vi "MyArchive.vi"(5 "archive filename":string, 6 "error in":errorcluster, 7 "archive mode":enum16{"direct", "append"}(ring), 8 "blocks to write":i32, 9 "ReadBuff refnum":refnum<file>) -> (0 "error out":errorcluster)   [LabVIEW 2013]
uses:
  My circular buffer info.ctl
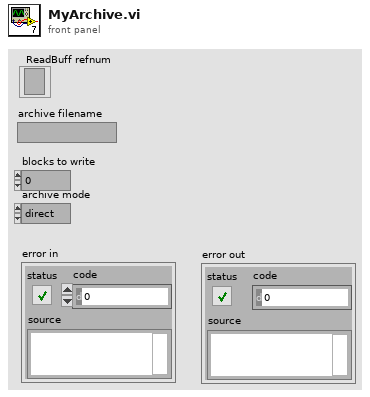
[diagram p1: front panel]
types:
  T1 = typedef "My circular buffer info.ctl" = cluster{"buff ref1":refnum<file>, "buff ref2":refnum<file>, "buffer1 path":path, "buffer2 path":path, "archive directory":path, "xml header":string, "num blocks  prior":i32, "num blocks after":i32, "blocks/event":i32, "samples/block":i32, "bytes/sample":i32, "number of channels":i32, "samples/block/channel":i32, "read buffer ref queue":refnum<queue>, "Event delay queue":refnum<queue>, "command queue":refnum<queue>}
  T2 = enum16{"open", "replace", "create", "open or create", "replace or create", "replace or create with confirmation"}
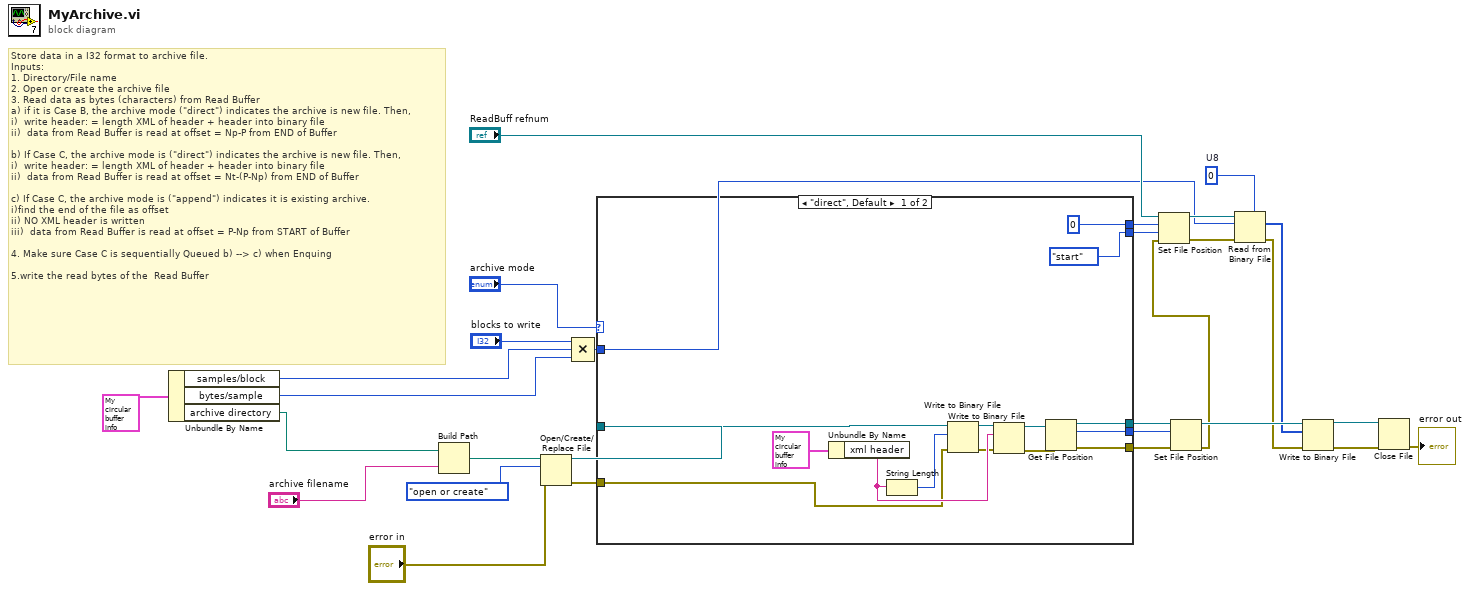
[diagram p0: block diagram]
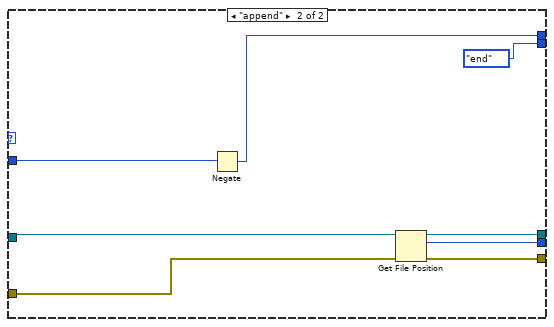
[diagram p2: hidden frame]
diagram:
  w16 = u8 0  # U8
  # "Store data in a I32 format to archive file.\nInputs:\n1. Directory/File name\n2. Open or create the archive file\n3. Read data as bytes (characters) from Read Buffer\na) if it is Case B, the archive mode (\"direct\") indicates the archive is new file. Then, \ni)  write header: = length XML of header + header into binary file\nii)  data from Read Buffer is read at offset = Np-P from END of Buffer\n\nb) If Case C, the archive mode is (\"direct\") indicates the archive is new file. Then, \ni)  write header: = length XML of header + header into binary file\nii)  data from Read Buffer is read at offset = Nt-(P-Np) from END of Buffer\n\nc) If Case C, the archive mode is (\"append\") indicates it is existing archive.  \ni)find the end of the file as offset\nii) NO XML header is written\niii)  data from Read Buffer is read at offset = P-Np from START of Buffer\n\n4. Make sure Case C is sequentially Queued b) --> c) when Enquing\n\n5.write the read bytes of the  Read Buffer"
  n1 = Unbundle By Name(T1 {"buff ref1"=refnum, "buff ref2"=refnum, "buffer1 path"=path "", "buffer2 path"=path "", "archive directory"=path "", "xml header"="", "num blocks  prior"=0, "num blocks after"=0, "blocks/event"=0, "samples/block"=0, "bytes/sample"=0, "number of channels"=0, "samples/block/channel"=0, "read buffer ref queue"=refnum, "Event delay queue"=refnum, "command queue"=refnum} ("My circular buffer info")) -> ("samples/block"=w22:i32, "bytes/sample"=w23:i32, "archive directory"=w28:path)
  n2 = Build Path(base path=w28, name or relative path="archive filename") -> (appended path=w26:path)
  n3 = Open/Create/Replace File(file path (use dialog)=w26, error in="error in", operation (0:open)=T2."open or create") -> (refnum out=w15:refnum<file>, error out=w7:errorcluster)  [unwired: 3 in, 1 out]
  n4 = Compound Arithmetic op=MULTIPLY("blocks to write", w22, w23) -> (w9:i32)
  n5 = case shown="\"direct\", Default" "archive mode" {
    tunnel: w9 -> [_ w51]
    tunnel: [0 w50] -> w20
    tunnel: [enum16{"start", "end", "current"}."start" ("from (0:start)") enum16{"start", "end", "current"}."end" ("from (0:start)")] -> w19
    tunnel: w15 -> [w41 w46]
    tunnel: [w36 w47] -> w14
    tunnel: [w35 w48] -> w13
    tunnel: w7 -> [w33 w45]
    tunnel: [w30 w44] -> w6
    frame "direct", Default {
      n6 = Unbundle By Name(T1 {"buff ref1"=refnum, "buff ref2"=refnum, "buffer1 path"=path "", "buffer2 path"=path "", "archive directory"=path "", "xml header"="", "num blocks  prior"=0, "num blocks after"=0, "blocks/event"=0, "samples/block"=0, "bytes/sample"=0, "number of channels"=0, "samples/block/channel"=0, "read buffer ref queue"=refnum, "Event delay queue"=refnum, "command queue"=refnum} ("My circular buffer info")) -> ("xml header"=w38:string)
      n7 = String Length(string=w38) -> (length=w40:i32)
      n8 = Write to Binary File(file (use dialog)=w41, data=w40, error in=w33) -> (refnum out=w39:refnum<file>, error out=w32:errorcluster)  [unwired: 3 in, 1 out]
      n9 = Write to Binary File(file (use dialog)=w39, data=w38, error in=w32) -> (refnum out=w37:refnum<file>, error out=w31:errorcluster)  [unwired: 3 in, 1 out]
      n10 = Get File Position(4:w31, 7:w37) -> (0:w30:errorcluster, 2:w35:i64, 3:w36:refnum<file>)
    }
    frame "append" {
      n11 = Negate(x=w51) -> (-x=w50:i32)
      n12 = Get File Position(4:w45, 7:w46) -> (0:w44:errorcluster, 2:w48:i64, 3:w47:refnum<file>)
    }
  }
  n13 = Set File Position(offset (in bytes) (0)=w13, refnum=w14, error in=w6) -> (refnum out=w12:refnum<file>, error out=w5:errorcluster)  [unwired: 1 in]
  n14 = Set File Position(offset (in bytes) (0)=w20, refnum="ReadBuff refnum", from (0:start)=w19, error in=w5) -> (refnum out=w17:refnum<file>, error out=w4:errorcluster)
  n15 = Read from Binary File(5:w16, 8:w4, 10:w9, 11:w17) -> (0:w3:errorcluster, 2:w11:u8[])  [unwired: 2 in, 2 out]
  n16 = Write to Binary File(file (use dialog)=w12, data=w11, error in=w3) -> (refnum out=w10:refnum<file>, error out=w2:errorcluster)  [unwired: 3 in, 1 out]
  n17 = Close File(refnum=w10, error in=w2) -> (error out=→"error out":errorcluster)  [unwired: 1 out]
